vi "PR Error Code.vi"() -> (0 "bErrorCode Out":bool[](array[boolean]))   [LabVIEW 2022 SP3, in "BS6006PRPLUS.lvlib"]
doc: "The function gets the error code of the pulser/receiver. \n\nextern \"C\" BS6006PRPLUS_API void __cdecl PR_ErrorCode(bool *bErrorCode);"
uses:
  BS6006PRPLUS.lvlib
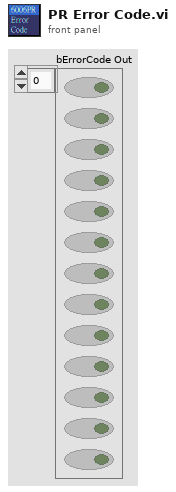
[diagram p1: front panel]
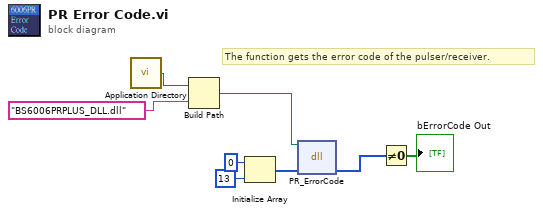
[diagram p0: block diagram]
diagram:
  # "The function gets the error code of the pulser/receiver."
  n1 = call <vilib>:"Application Directory.vi"() -> ("Application Directory"=w3:path)
  n2 = Build Path(base path=w3, name or relative path="BS6006PRPLUS_DLL.dll") -> (appended path=w1:path)
  n3 = Initialize Array(u8 0 ("element"), 13 ("dimension size")) -> (w4:u8[])
  n4 = dll-call lib="E:/Broadsound_Program/PulserReceiver/6006PR PLUS/API/DLL/LabVIEW 15/VIs/BS6006PRPLUS_DLL.dlls" fn="PR_ErrorCode"(path in=w1, "bErrorCode"=w4) -> ("bErrorCode"=w8:u8[])  [unwired: 3 in, 2 out]
  n5 = Not Equal To 0?(x=w8) -> (x != 0?=→"bErrorCode Out":bool[])
